vi "Analog Input - Filtering.vi"() -> ()   [LabVIEW 2022 SP3]
doc: "This example demonstrates how to utilize filtering properties of C Series and FieldDAQ devices.\n\nFor instructions on how to connect your signals to the DAQ device, refer to your device documentation."
uses:
  <vilib>/Utility/error.llb/DialogType.ctl
  <vilib>/DAQmx/read.llb/DAQmx Read (Analog 1D Wfm NChan NSamp).vi
  <vilib>/DAQmx/create/channels.llb/DAQmx Create Channel (AI-Voltage-Basic).vi
  <vilib>/DAQmx/create/channels.llb/DAQmx Create Channel (AI-Current-Basic).vi
  <vilib>/DAQmx/create/channels.llb/DAQmx Create Channel (AI-Strain-Strain Gage).vi
  <vilib>/DAQmx/configure/timing.llb/DAQmx Timing (Sample Clock).vi
  <vilib>/DAQmx/configure/task.llb/DAQmx Configure Logging (TDMS).vi
  <vilib>/DAQmx/configure/trigger.llb/DAQmx Start Trigger (Digital Edge).vi
  <vilib>/DAQmx/configure/trigger.llb/DAQmx Start Trigger (Time).vi
  <vilib>/DAQmx/configure/trigger.llb/DAQmx Start Trigger (Analog Edge).vi
  <vilib>/DAQmx/miscellaneous.llb/DAQmx Fill In Error Info.vi
  <resource>/objmgr/daqmx.rc
panel:
  in  "Task Type":T1(tab)
  in  "Max Voltage":dbl=5.0
  in  "Min Voltage":dbl=-5.0
  in  "units":i32(ring)=10348 items=["Volts"=10348, "From Custom Scale"=10065]
  in  "Max Current":dbl=0.01 format="%0.5f"
  in  "Min Current":dbl=-0.01 format="%0.5f"
  in  "shunt resistor location":i32(ring)=-1 items=["default"=-1, "Internal"=10200, "External"=10167]
  in  "external shunt resistor value":dbl=249.0 format="%0.2f"
  in  "Units":i32(ring)=10342 items=["Amps"=10342, "From Custom Scale"=10065]
  in  "Units":i32(ring)=10299 items=["Amps"=10299, "From Custom Scale"=10065]
  in  "Min Input":dbl=-0.001 format="%#_13g"
  in  "Max Input":dbl=0.001 format="%0.7f"
  in  "bridge information":T2={"strain configuration"=10183, "lead wire resistance"=0.0, "initial bridge voltage"=0.0, "voltage excitation source"=10200, "voltage excitation value"=2.5} {"strain configuration" items=["Full Bridge I"=10183, "Full Bridge II"=10184, "Full Bridge III"=10185, "Half Bridge I"=10188, "Half Bridge II"=10189, "Quarter Bridge I"=10271, "Quarter Bridge II"=10272]; "voltage excitation source" items=["Internal"=10200, "External"=10167, "None"=10230]}
  in  "strain gage information":T3={"gage factor"=2.0, "nominal gage resistance"=350.0, "poisson ratio"=0.3}
  out "Actual Filter Response":i32(ring)=16152 items=["Comb"=16152, "Bessel"=16153, "Brickwall"=16155, "Butterworth"=16076]
  in  "Filter Response":i32(ring)=16152 items=["Comb"=16152, "Bessel"=16153, "Brickwall"=16155, "Butterworth"=16076]
  out "Actual Filter Order":u32
  in  "Filter Order":u32=1
  out "Actual Filter Frequency":dbl
  in  "Filter Frequency":dbl=1000.0
  in  "Filter":enum16{"No Filtering", "Filtering"}(ring)=enum."Filtering"
  in  "Trigger Type":T4(tab)
  in  "Digital Start Trigger Edge":i32(ring)=10280 caption="Edge" items=["Rising"=10280, "Falling"=10171]
  in  "Digital Start Trigger Source":tag="/Dev1/PFI0" caption="Source"
  in  "Digital Pause Trigger Pause When":i32(ring)=10192 caption="Pause When" items=["High"=10192, "Low"=10214]
  in  "Digital Pause Trigger Source":tag="/Dev1/PFI0" caption="Source"
  in  "Analog Start Trigger Level":dbl caption="Level" format="%0.2f"
  in  "Analog Start Trigger Hysteresis":dbl caption="Hysteresis" format="%.2f"
  in  "Analog Start Trigger Slope":i32(ring)=10280 caption="Slope" items=["Rising"=10280, "Falling"=10171]
  in  "Analog Start Trigger Source":string="APFI0" caption="Source"
  in  "Analog Pause Trigger Source":string="APFI0" caption="Source"
  in  "Analog Pause Trigger Pause When":i32(ring)=10093 caption="Pause When" items=["Above Level"=10093, "Below Level"=10107]
  in  "Analog Pause Trigger Level":dbl caption="Level" format="%.2f"
  in  "When":timestamp
  in  "Select Time\nManually":bool
  in  "Stop":bool
  out "Waveform Graph":waveform(dbl)[](graph)=[{"t0"=timestamp(3628080175.5424995 s since 1904-01-01), "dt"=0.001, "Y"=[3.339760288462809, 3.363838943366331, 3.325639202680636, 3.702971017001809, 3.512829555662086, 3.3596366813003664, 3.3189636922531425, 3.588697902104663, 3.5297855135871075, 3.54184502093738, 3.4076228655680363, 3.4210707499358772, 3.3263140184868494, 3.355484465382709, 3.641175324584978, 3.631611667082567, 3.3205813129177972, 3.518289429003267, 3.4664077171270016, 3.314751743835892, 3.5647596992947785, 3.5382207111647745, 3.5375103787371818, 3.582984569238182, 3.4814958236458295, 3.5707636226998205, 3.4453318311219405, 3.2571986732820486, 3.4674909740790807, 3.5187559882568453, 3.2498935500210067, 3.4613288402697115, 3.3491140750207045, 3.4501846931159053, 3.496503210570613, 3.3587100203607334, 3.4416042002689577, 3.5185106006909495, 3.474216530654882, 3.192979778651997, 3.196807501801595, 3.39810441103829, 3.36649300361852, 3.3714330427740533, 3.190588864276394, 3.4819930563451447, 3.5523740847845655, 3.15925997543578, 3.404379552279322, 3.386170826254727, 3.4579660619818107, 3.160806562857676, 3.1445447934414386, 3.256562602880977, 3.3726712813466984, 3.3737561526906585, 3.2735895940487576, 3.423548841473048, 3.5053371629428605, 3.4313205239876683, 3.5034386380909304, 3.431988882226358, 3.2884888167175212, 3.318041874489152, 3.1426898571702924, 3.30339772573757, 3.3307665112943527, 3.4547243630849773, 3.3303193247433454, 3.1832240085157593, 3.27536542511774, 3.2511317885936517, 3.302716452363833, 3.417473884825247, 3.246101343492789, 3.116005573771008, 3.3526802666855975, 3.243129248040064, 3.358109466581041, 3.3350785520082185, 3.370653291495582, 3.386404913077457, 3.286189922679129, 3.1814368767036103, 3.126229517552705, 3.0344707118264957, 3.2755978975485887, 3.0140841711545763, 3.338123295095583, 3.381535907164683, 3.3057224500460562, 3.383306895058023, 3.1254901260712558, 3.3383719114452406, 3.0101030807762936, 3.086634942281918, 3.0471614464021974, 3.2640356228976315, 3.1273434479505213, 3.196124614035977], "attributes"=variant("NI_ChannelName"=variant(string "cDAQ1Mod4/ai0"), "NI_UnitDescription"=variant(string "Volts"))}]
  in  "TDMS File Path":path
  in  "Number of Samples":i32=100
  in  "Sample Rate":dbl=1000.0
  in  "Sample Clock Source":tag="OnboardClock"
  in  "Terminal Configuration":i32(ring)=-1 items=["default"=-1, "RSE"=10083, "NRSE"=10078, "Differential"=10106, "Pseudodifferential"=12529]
  in  "Physical Channel":tag="cDAQ1Mod1/ai0"
  out "Actual Sample Rate":dbl=1000.0 format="%0.2f"
  in  "Logging Mode":i32(ring)=10231 items=["Off"=10231, "Log and Read"=15842]
  # "Channel Settings"
  # "Acquired Data"
  # "Timing Settings"
  # "Trigger Settings"
  # "Logging Settings"
  # "Task Type Settings"
  # "Filtering Settings"
  # "Use this tab control to set task \nconfigurations for your measurement.\nStart by selecting the tab that \ncorresponds to your measurment type\nthen configure settings appropriately"
  # "To enable triggers, select a tab above, and configure the settings.\n\nNot all hardware supports all trigger types. Refer to your device documentation for more information."
  # "This trigger type is not supported in continuous sample timing. \n\nRefer to your device documentation for more information on which triggers are supported."
  # "This trigger type is not supported in continuous sample timing. \n\nRefer to your device documentation for more information on which triggers are supported."
  # "If time is not manually set, task will begin after 10 seconds"
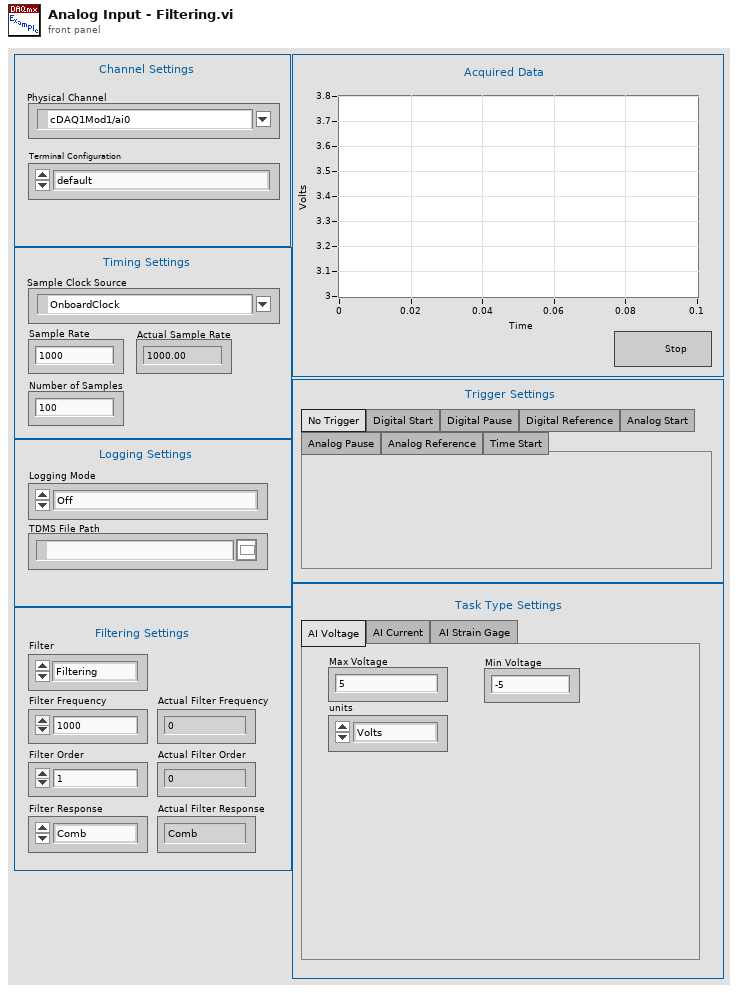
[diagram p1: front panel]
types:
  T1 = enum32{"AI Voltage", "AI Current", "AI Strain Gage "}
  T2 = cluster{"strain configuration":i32, "lead wire resistance":dbl, "initial bridge voltage":dbl, "voltage excitation source":i32, "voltage excitation value":dbl}
  T3 = cluster{"gage factor":dbl, "nominal gage resistance":dbl, "poisson ratio":dbl}
  T4 = enum32{"No Trigger", "Digital Start", "Digital Pause", "Digital Reference", "Analog Start", "Analog Pause", "Analog Reference", "Time Start"}
  T5 = typedef "DialogType.ctl" = u16
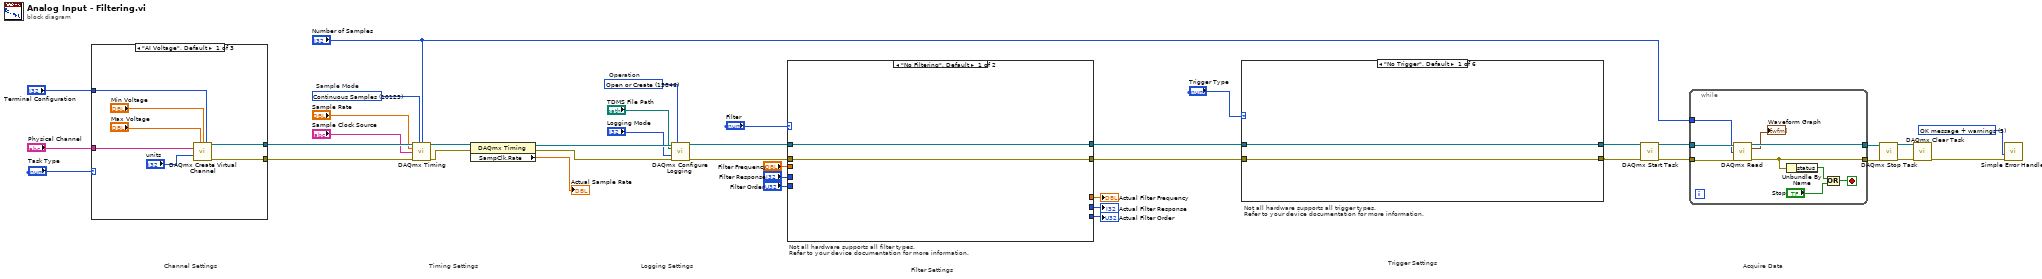
[diagram p0: block diagram]
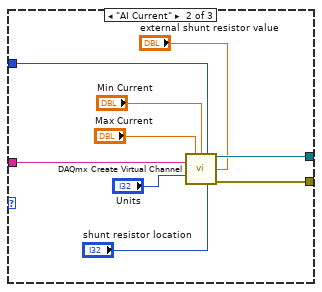
[diagram p2: hidden frame]
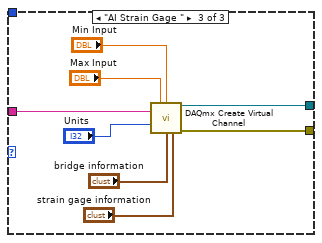
[diagram p3: hidden frame]
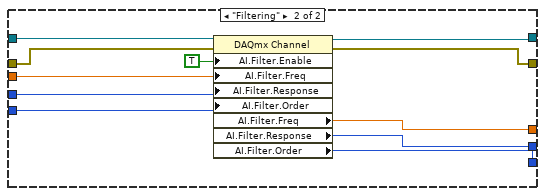
[diagram p4: hidden frame]
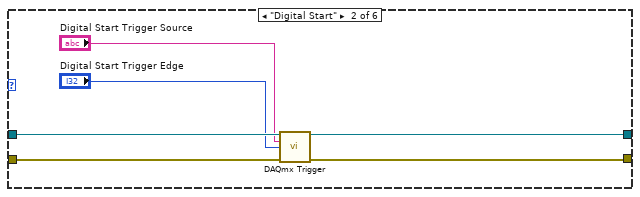
[diagram p5: hidden frame]
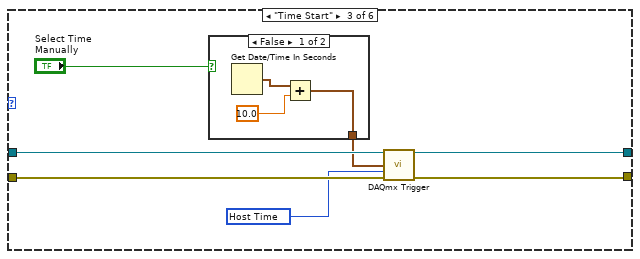
[diagram p6: hidden frame]
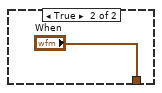
[diagram p7: hidden frame]
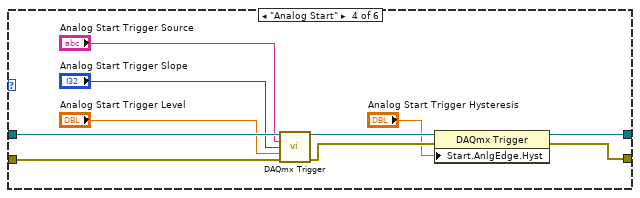
[diagram p8: hidden frame]
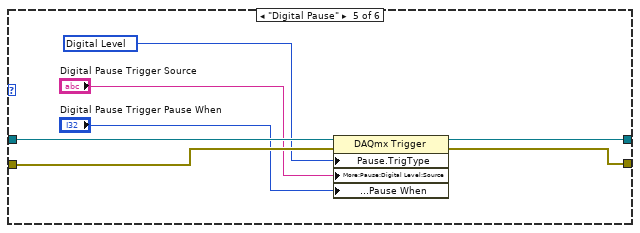
[diagram p9: hidden frame]
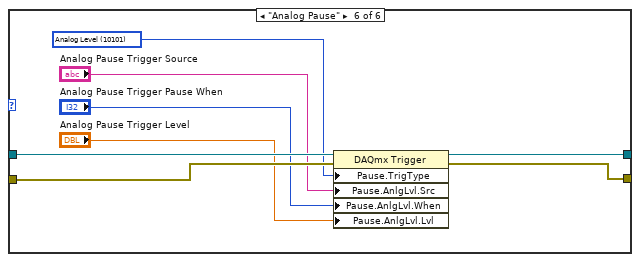
[diagram p10: hidden frame]
diagram:
  w18 = T5 3 items=["no dialog", "OK message", "continue or stop message", "OK message + warnings", "continue/stop + warnings"] ("type of dialog (OK msg:1)")
  w32 = 15846 items=["Open"=10437, "Open or Create"=15846, "Create or Replace"=15847, "Create"=15848]  # Operation
  w37 = 10123 items=["Finite Samples"=10178, "Continuous Samples"=10123, "Hardware Timed Single Point"=12522]  # Sample Mode
  # "Filter Settings"
  # "Not all hardware supports all filter types.\nRefer to your device documentation for more information."
  # "Trigger Settings"
  # "Not all hardware supports all trigger types.\nRefer to your device documentation for more information."
  # "Acquire Data"
  # "Timing Settings"
  # "Channel Settings"
  # "Logging Settings"
  n1 = case shown="\"AI Voltage\", Default" "Task Type" {
    tunnel: [w46 w55 w62] -> w36
    tunnel: [w45 w54 w63] -> w35
    tunnel: "Physical Channel" -> [w42 w53 w61]
    tunnel: "Terminal Configuration" -> [w41 w52 _]
    frame "AI Voltage", Default {
      n2 = call-poly <vilib>:"DAQmx Create Virtual Channel.vi"("maximum value"="Max Voltage", "minimum value"="Min Voltage", "input terminal configuration"=w41, "physical channels"=w42, "units"="units") -> ("task out"=w45:refnum<k21>, "error out"=w46:errorcluster)  [unwired: 9 in]
    }
    frame "AI Current" {
      n3 = call-poly <vilib>:"DAQmx Create Virtual Channel.vi"("maximum value"="Max Current", "minimum value"="Min Current", "input terminal configuration"=w52, "physical channels"=w53, "external shunt resistor value"="external shunt resistor value", "units"="Units", "shunt resistor location"="shunt resistor location") -> ("task out"=w54:refnum<k21>, "error out"=w55:errorcluster)  [unwired: 7 in]
    }
    frame "AI Strain Gage " {
      n4 = call-poly <vilib>:"DAQmx Create Virtual Channel.vi"("maximum value"="Max Input", "minimum value"="Min Input", "physical channels"=w61, "units"="Units", "bridge information"="bridge information", "strain gage information"="strain gage information") -> ("task out"=w63:refnum<k21>, "error out"=w62:errorcluster)  [unwired: 8 in]
    }
  }
  n5 = call-poly <vilib>:"DAQmx Timing.vi"("task/channels in"=w35, "sample mode"=w37, "samples per channel"="Number of Samples", "rate"="Sample Rate", "source"="Sample Clock Source", "error in"=w36) -> ("task out"=w39:refnum<k21>, "error out"=w38:errorcluster)  [unwired: 8 in]
  n6 = property class="DAQmx Timing"(reference=w39, error in=w38) -> (reference out=w34:refnum<k21>, error out=w33:errorcluster, "SampClk.Rate"=→"Actual Sample Rate":dbl)
  n7 = call-poly <vilib>:"DAQmx Configure Logging.vi"("task/channels in"=w34, "operation"=w32, "file path"="TDMS File Path", "logging mode"="Logging Mode", "error in"=w33) -> ("task out"=w13:refnum<k21>, "error out"=w12:errorcluster)  [unwired: 9 in]
  n8 = case shown="\"No Filtering\", Default" "Filter" {
    tunnel: w13 -> [w65 w76]
    tunnel: w12 -> [w64 w73]
    tunnel: [w65 w75] -> w11
    tunnel: [w64 w74] -> w10
    tunnel: "Filter Frequency" -> [_ w72]
    tunnel: "Filter Order" -> [_ w69]
    tunnel: [_ w68] -> w7
    tunnel: [_ w66] -> w6
    tunnel: [_ w67] -> w4
    tunnel: "Filter Response" -> [_ w70]
    frame "No Filtering", Default {
    }
    frame "Filtering" {
      n9 = property class="DAQmx Channel"(reference=w76, error in=w73, "AI.Filter.Enable"=TRUE, "AI.Filter.Freq"=w72, "AI.Filter.Response"=w70, "AI.Filter.Order"=w69) -> (reference out=w75:refnum<k21>, error out=w74:errorcluster, "AI.Filter.Freq"=w68:dbl, "AI.Filter.Response"=w67:i32, "AI.Filter.Order"=w66:u32)
    }
  }
  "Actual Filter Frequency" <- w7
  "Actual Filter Order" <- w6
  "Actual Filter Response" <- w4
  n10 = case shown="\"No Trigger\", Default" "Trigger Type" {
    tunnel: w11 -> [w78 w84 w91 w105 w112 w120]
    tunnel: w10 -> [w77 w83 w90 w104 w109 w117]
    tunnel: [w78 w82 w89 w102 w111 w119] -> w15
    tunnel: [w77 w81 w88 w101 w110 w118] -> w16
    frame "No Trigger", Default {
    }
    frame "Digital Start" {
      n11 = call-poly <vilib>:"DAQmx Trigger.vi"("task/channels in"=w84, "source"="Digital Start Trigger Source", "edge"="Digital Start Trigger Edge", "error in"=w83) -> ("task out"=w82:refnum<k21>, "error out"=w81:errorcluster)  [unwired: 10 in]
    }
    frame "Time Start" {
      w87 = 16126 items=["Host Time"=16126, "I/O Device Time"=16127] ("timescale")
      n12 = case shown="False" "Select Time\nManually" {
        tunnel: [w92 "When"] -> w85
        frame False {
          n13 = Get Date/Time In Seconds() -> (seconds since 1Jan1904=w94:timestamp)
          n14 = Add(x=w94, y=10.0) -> (x+y=w92:timestamp)
        }
        frame True {
        }
      }
      n15 = call-poly <vilib>:"DAQmx Trigger.vi"("task/channels in"=w91, "when"=w85, "timescale"=w87, "error in"=w90) -> ("task out"=w89:refnum<k21>, "error out"=w88:errorcluster)  [unwired: 10 in]
    }
    frame "Analog Start" {
      n16 = call-poly <vilib>:"DAQmx Trigger.vi"("task/channels in"=w105, "source"="Analog Start Trigger Source", "slope"="Analog Start Trigger Slope", "level"="Analog Start Trigger Level", "error in"=w104) -> ("task out"=w100:refnum<k21>, "error out"=w99:errorcluster)  [unwired: 9 in]
      n17 = property class="DAQmx Trigger"(reference=w100, error in=w99, "Start.AnlgEdge.Hyst"="Analog Start Trigger Hysteresis") -> (reference out=w102:refnum<k21>, error out=w101:errorcluster)
    }
    frame "Digital Pause" {
      w108 = 10152 items=["Analog Level"=10101, "Analog Window"=10103, "Digital Level"=10152, "Digital Pattern"=10398, "None"=10230] ("Pause.TrigType")
      n18 = property class="DAQmx Trigger"(reference=w112, error in=w109, "Pause.TrigType"=w108, "More:Pause:Digital Level:Source"="Digital Pause Trigger Source", "More:Pause:Digital Level:Pause When"="Digital Pause Trigger Pause When") -> (reference out=w111:refnum<k21>, error out=w110:errorcluster)
    }
    frame "Analog Pause" {
      w116 = 10101 items=["Analog Level"=10101, "Analog Window"=10103, "Digital Level"=10152, "Digital Pattern"=10398, "None"=10230] ("Pause.TrigType")
      n19 = property class="DAQmx Trigger"(reference=w120, error in=w117, "Pause.TrigType"=w116, "Pause.AnlgLvl.Src"="Analog Pause Trigger Source", "Pause.AnlgLvl.When"="Analog Pause Trigger Pause When", "Pause.AnlgLvl.Lvl"="Analog Pause Trigger Level") -> (reference out=w119:refnum<k21>, error out=w118:errorcluster)
    }
  }
  n20 = call <vilib>:"DAQmx Start Task.vi"("task/channels in"=w15, "error in"=w16) -> ("task out"=w31:refnum<k21>, "error out"=w30:errorcluster)  [unwired: 12 in]
  n21 = while {
    tunnel: w31 -> [w129]
    tunnel: w30 -> [w128]
    tunnel: [w127] -> w22
    tunnel: [w124] -> w21
    tunnel: "Number of Samples" -> [w121]
    stop <- w122 stop-if-true
    n22 = call-poly <vilib>:"DAQmx Read.vi"("task/channels in"=w129, "number of samples per channel"=w121, "error in"=w128) -> ("task out"=w127:refnum<k21>, "data"=→"Waveform Graph":waveform(dbl)[], "error out"=w124:errorcluster)  [unwired: 10 in]
    n23 = Unbundle By Name(w124) -> ("status"=w123:bool)
    n24 = Or(x=w123, y="Stop") -> (x .or. y?=w122:bool)
  }
  n25 = call <vilib>:"DAQmx Stop Task.vi"("task/channels in"=w22, "error in"=w21) -> ("task out"=w19:refnum<k21>, "error out"=w20:errorcluster)  [unwired: 12 in]
  n26 = call <vilib>:"DAQmx Clear Task.vi"("task in"=w19, "error in"=w20) -> ("error out"=w29:errorcluster)  [unwired: 13 in]
  n27 = call <vilib>:"Simple Error Handler.vi"("type of dialog (OK msg:1)"=w18, "error in (no error)"=w29) -> ()  [unwired: 3 in, 5 out]
